vi "Result_Test.vi"(8 "error in (no error)":errorcluster caption="entrée d'erreur (pas d'erreur)", 11 "Flash_Jlink en entrée":refnum<class "Flash_STM32.lvclass">) -> (0 "error out":errorcluster caption="sortie d'erreur", 3 "Flash_Jlink en sortie":refnum<class "Flash_STM32.lvclass">)   [LabVIEW 2020, in "Library Test.lvlib" / "Flash_STM32.lvclass"]
uses:
  Flash_STM32.lvclass
  C:/Users/ngarcin/OneDrive - Altyor/Standard TB/Class/Test/Test (Default)/Test (Default).lvclass
  Test_Without_Instr/Test_Without_Inst.lvclass
  Flash_STM32.lvclass/Flash_STM32.ctl
panel:
  out "standard output":string caption="sortie standard"
  out "Ok":bool
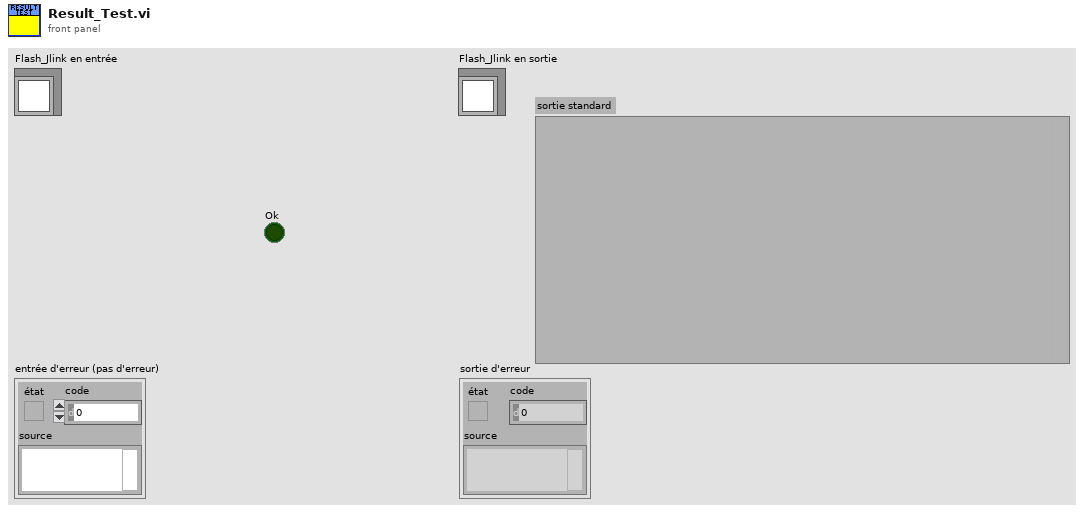
[diagram p1: front panel]
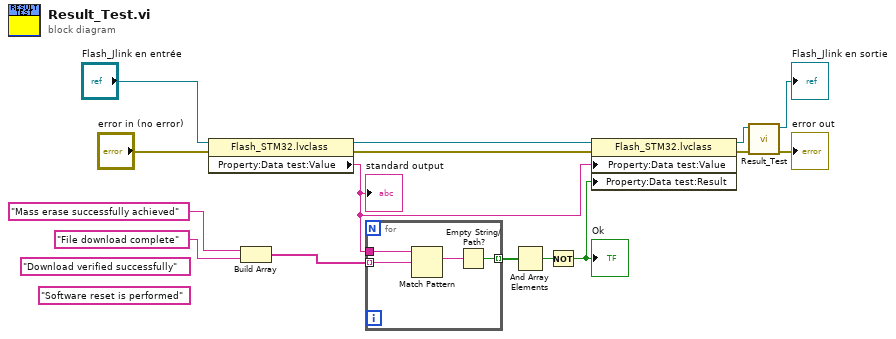
[diagram p0: block diagram]
diagram:
  (unwired) "Software reset is performed" ("expression régulière")
  (unwired) "Download verified successfully" ("expression régulière")
  n1 = property class="Flash_STM32.lvclass"(reference="Flash_Jlink en entrée", error in="error in (no error)") -> (reference out=w8:refnum<class "Flash_STM32.lvclass">, error out=w10:errorcluster, "Property:Data test:Value"=w7:string)
  "standard output" <- w7
  n2 = Build Array("Mass erase successfully achieved" ("expression régulière"), "File download complete" ("expression régulière")) -> (w5:string[])
  n3 = for {
    tunnel: w7 -> [w18]
    tunnel: [w17] -> w4 mode=indexing
    tunnel: w5 -> [w16] mode=indexing
    n4 = Match Pattern(string=w18, regular expression=w16) -> (match substring=w19:string)  [unwired: 1 in, 3 out]
    n5 = Empty String/Path?(string/path=w19) -> (empty?=w17:bool)
  }
  n6 = And Array Elements(Boolean array=w4) -> (logical AND=w3:bool)
  n7 = Not(x=w3) -> (.not. x?=w2:bool)
  "Ok" <- w2
  n8 = property class="Flash_STM32.lvclass"(reference=w8, error in=w10, "Property:Data test:Value"=w7, "Property:Data test:Result"=w2) -> (reference out=w12:refnum<class "Flash_STM32.lvclass">, error out=w15:errorcluster)
  n9 = call-parent "Result_Test.vi"("error in (no error)"=w15, "Test_Without_Inst en entrée"=w12) -> ("error out"=→"error out":errorcluster, "Test_Without_Inst en sortie"=→"Flash_Jlink en sortie":refnum<class "Flash_STM32.lvclass">)  [unwired: 8 in]
